vi "load_project.vi"(7 "lv-builder in":refnum<class "lv-builder.lvclass">, 8 "error in (no error)":errorcluster, 11 "project_file":path) -> (0 "error out":errorcluster, 1 "config":T3, 2 "lv-builder out":refnum<class "lv-builder.lvclass">, 3 "build_spec_info []":T1[](array[typedef]))   [LabVIEW 2015, in "lv-build-interface.lvlib"]
uses:
  lv-build-interface.lvlib
  lv-builder/class/lv-builder.lvclass
  lv-build/public/_controls/configuration.ctl
  lv-build/public/_controls/build_specification.ctl
  lv-build/public/_controls/build_type.ctl
  lv-build/lv-build.lvlib
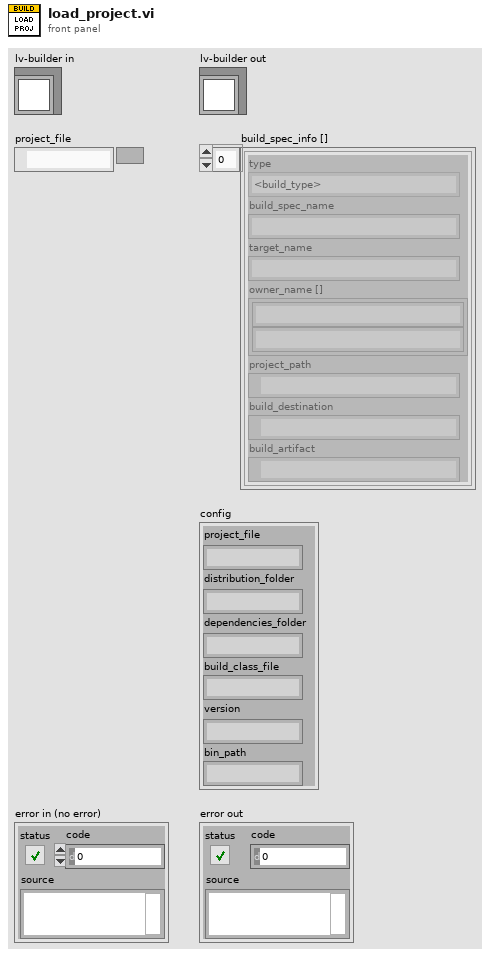
[diagram p1: front panel]
types:
  T1 = typedef "lv-build.lvlib/build_specification.ctl" = cluster{"type":T2, "build_spec_name":string, "target_name":string, "owner_name []":string[], "project_path":path, "build_destination":path, "build_artifact":path}
  T2 = typedef "lv-build.lvlib/build_type.ctl" = enum16{"<build_type>", "application_pc", "application_rt", "installer", "llb", "lvlibp", "zip", "fpga", "<null>"}
  T3 = typedef "lv-build.lvlib/configuration.ctl" = cluster{"project_file":string, "distribution_folder":string, "dependencies_folder":string, "build_class_file":string, "version":string, "bin_path":string}
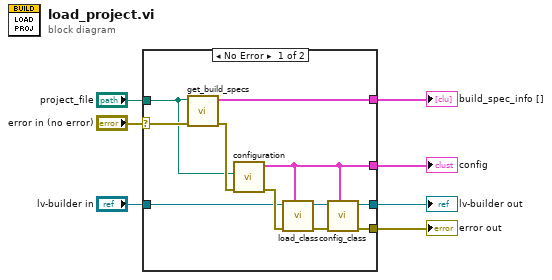
[diagram p0: block diagram]
diagram:
  n1 = case shown="No Error" "error in (no error)" {
    selector: "error in (no error)" -> [w15 w20]
    tunnel: [w16 _] -> w7
    tunnel: [w10 _] -> w5
    tunnel: [w12 w20] -> w4
    tunnel: [w11 w19] -> w3
    tunnel: "lv-builder in" -> [w14 w19]
    tunnel: "project_file" -> [w8 _]
    frame No Error {
      n2 = call "get_build_specs.vi"("error in (no error)"=w15, "project path"=w8) -> ("error out"=w17:errorcluster, "build_spec_info []"=w16:T1[])  [unwired: 8 in]
      n3 = call "configuration.vi"("error in (no error)"=w17, "project_file"=w8) -> ("error out"=w18:errorcluster, "config out"=w10:T3)  [unwired: 8 in]
      n4 = call "load_class.vi"("config in"=w10, "error in (no error)"=w18, "lv-builder in"=w14) -> ("error out"=w9:errorcluster, "lv-builder out"=w13:refnum<class "lv-builder.lvclass">)  [unwired: 7 in]
      n5 = call "config_class.vi"("config in"=w10, "error in (no error)"=w9, "lv-builder in"=w13) -> ("error out"=w12:errorcluster, "lv-builder out"=w11:refnum<class "lv-builder.lvclass">)  [unwired: 7 in]
    }
    frame Error {
    }
  }
  "lv-builder out" <- w3
  "error out" <- w4
  "config" <- w5
  "build_spec_info []" <- w7
